vi "Calibration AE.vi"(7 "Command":T1, 8 "error in (no error)":errorcluster, 11 "Inst Details In":string[][](array[string])) -> (0 "error out":errorcluster, 2 "Calibration Due Msg?":string[](array[string]), 3 "Inst Details Out":string[][](array[string]))   [LabVIEW 2016, in "Calibration.lvlib"]
uses:
  Calibration.lvlib
  Calibration Command.ctl
  User Interface/Create Path Command.ctl
  User Interface/User Interface.lvlib
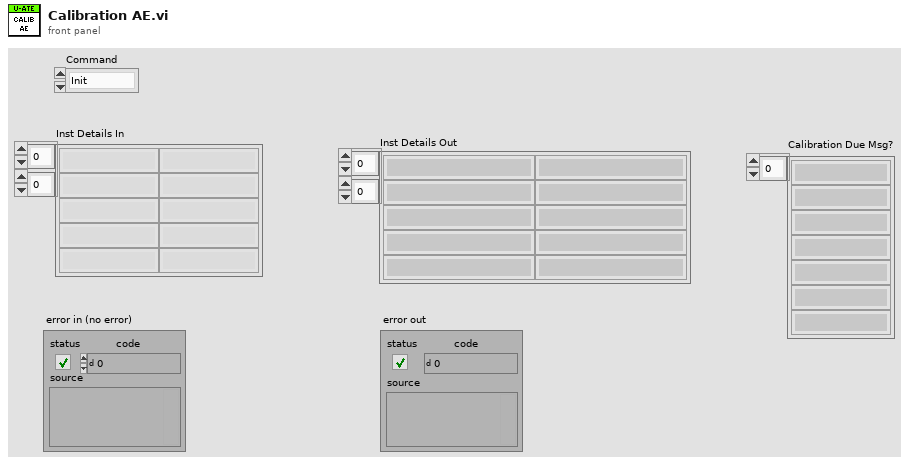
[diagram p1: front panel]
types:
  T1 = typedef "Calibration.lvlib/Calibration Command.ctl" = enum16{"Init", "Read", "Write", "Check Calibration", "Close"}
  T2 = typedef "User Interface.lvlib/Create Path Command.ctl" = enum16{"Authentication", "Hardware", "Configuration", "Calibration", "Instrument", "Test Description", "Data", "Report", "Action log", "Error Log"}
  T3 = enum16{"open", "open or create", "create or replace", "create", "open (read-only)"}
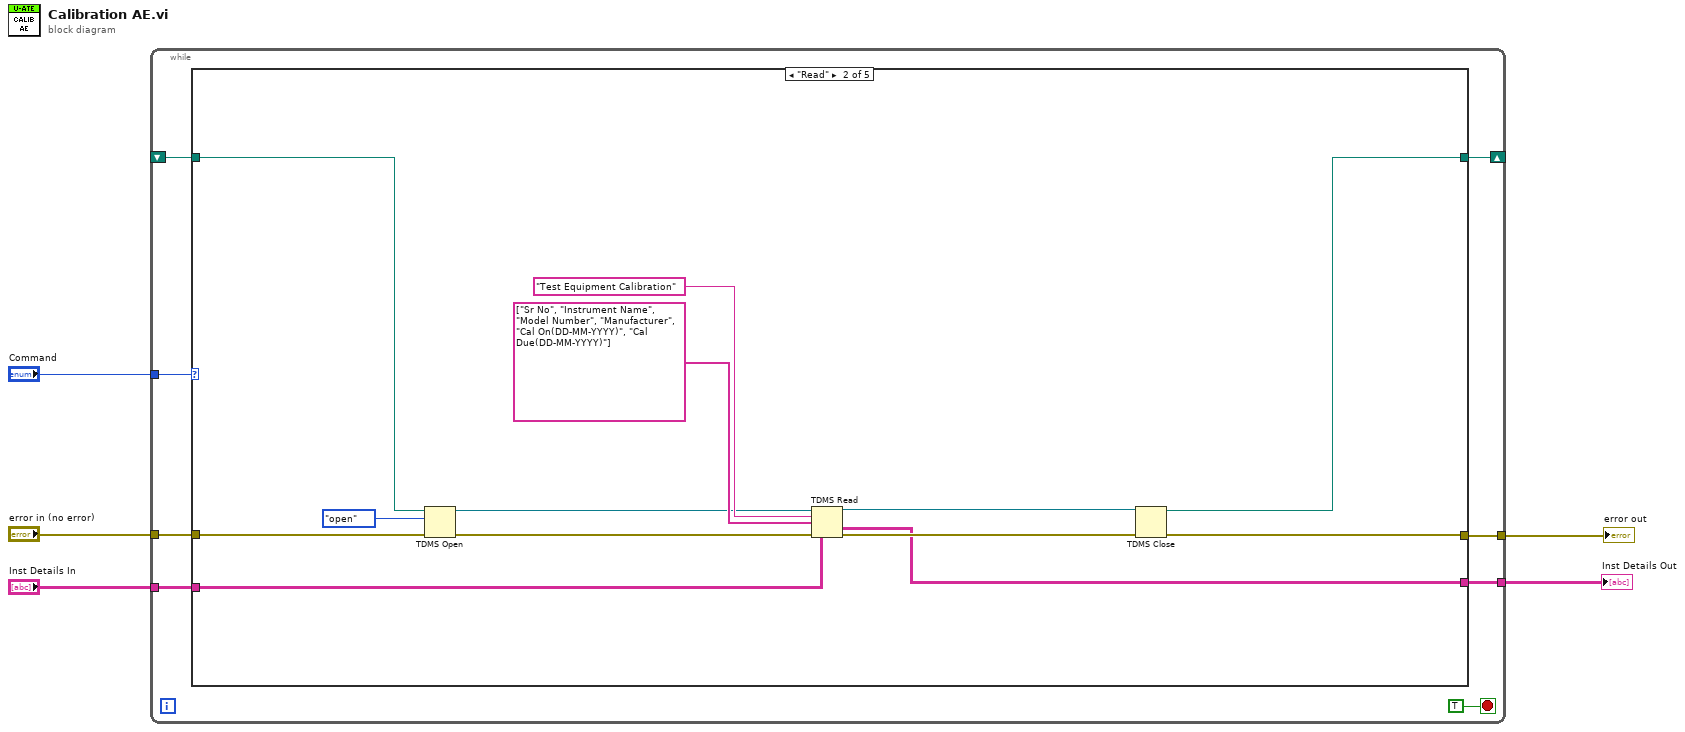
[diagram p0: block diagram]
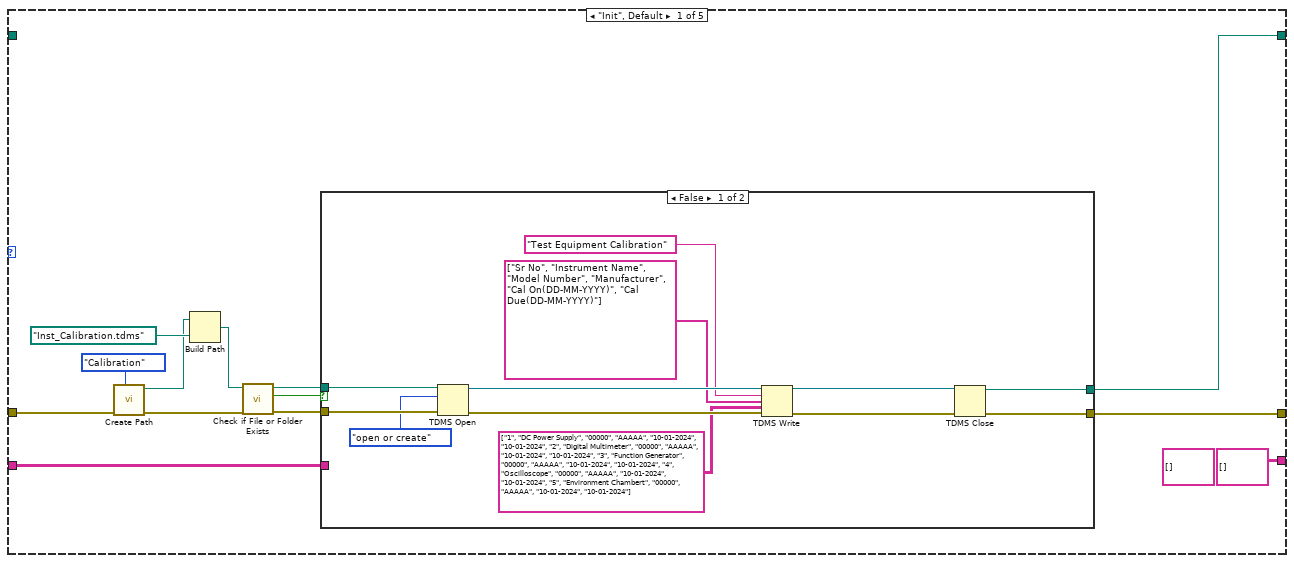
[diagram p2: hidden frame]
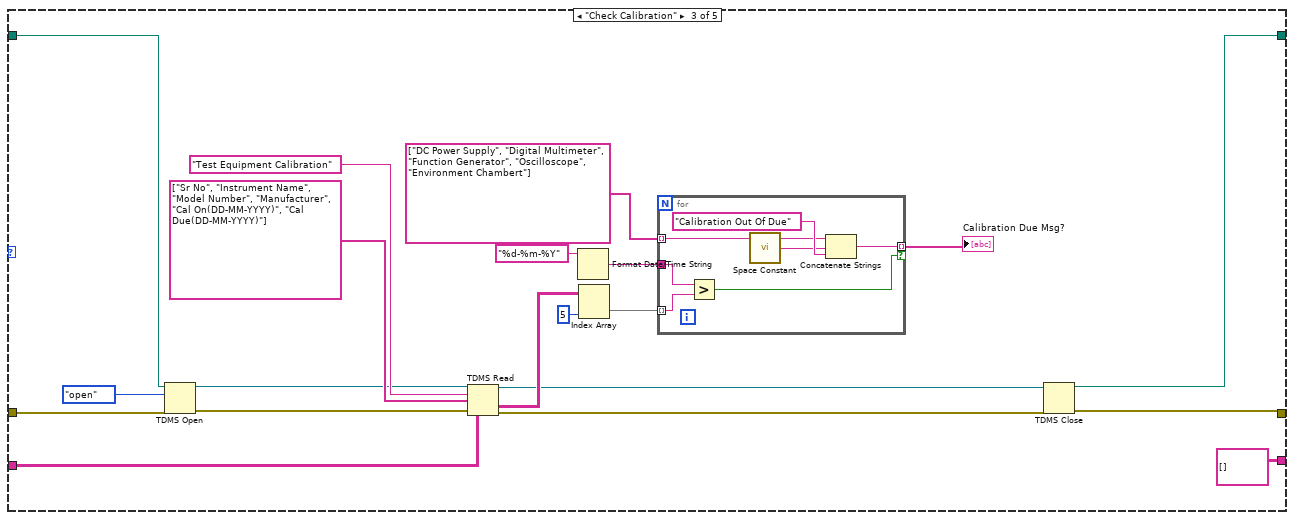
[diagram p4: hidden frame]
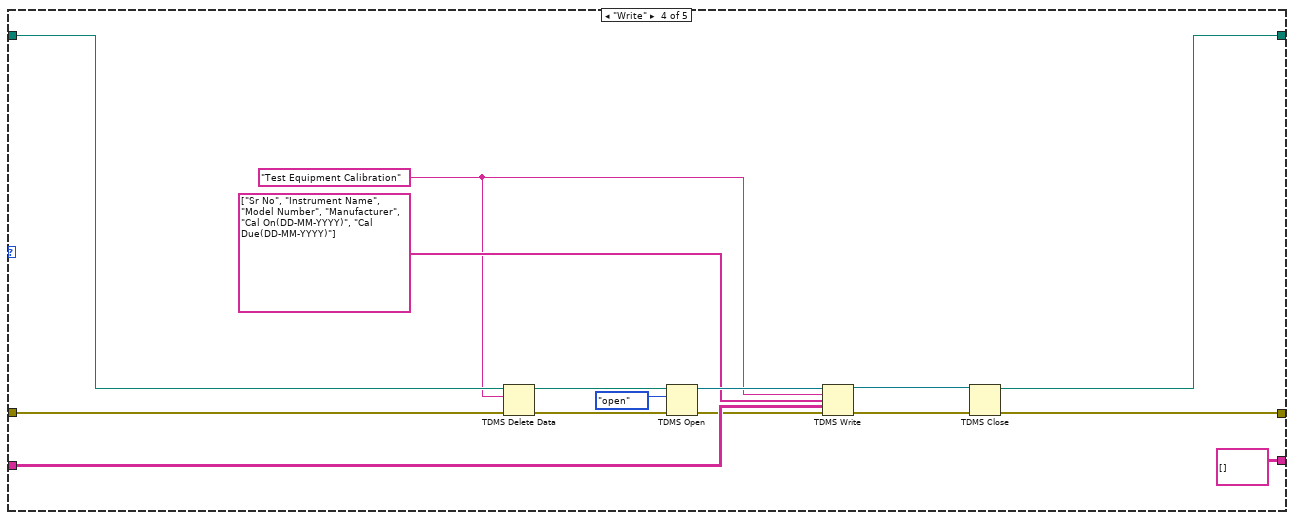
[diagram p5: hidden frame]
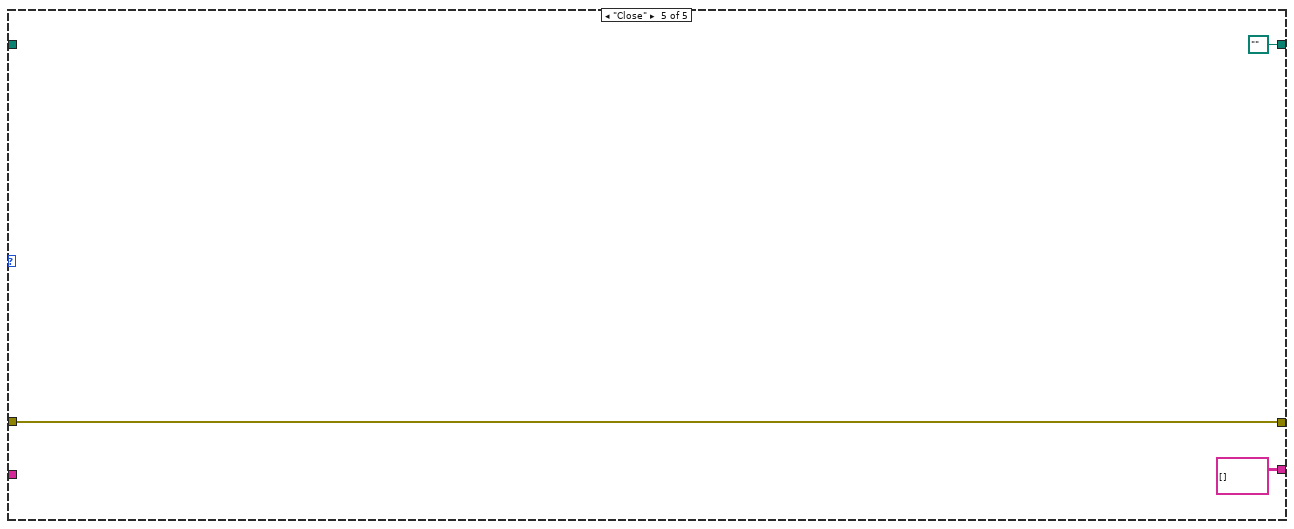
[diagram p6: hidden frame]
diagram:
  n1 = while {
    tunnel: "error in (no error)" -> [w12]
    tunnel: "Inst Details In" -> [w10]
    tunnel: [w9] -> w2
    tunnel: "Command" -> [w11]
    tunnel: [w8] -> w1
    shift-right: [w7] -> _
    shift-left: _ -> [w6]
    stop <- TRUE stop-if-true
    n2 = case shown="\"Read\"" w11 {
      tunnel: w12 -> [w26 w53 w72 w87 w98]
      tunnel: w10 -> [w20 w50 w68 w94 _]
      tunnel: [w19 w43 w56 w90 w98] -> w9
      tunnel: [string[][] [] ("Inst Details In") w48 string[][] [] ("Inst Details In") string[][] [] ("Inst Details In") string[][] [] ("Inst Details In")] -> w8
      tunnel: [w17 w41 w55 w88 path "" ("file path out")] -> w7
      tunnel: w6 -> [_ w46 w71 w86 _]
      frame "Init", Default {
        (unwired) string[][] [] ("Inst Details In")
        n3 = call "Create Path.vi"("Path Command"=Create_Path_Command."Calibration", "error in (no error)"=w26) -> ("error out"=w16:errorcluster, "created path"=w14:path)  [unwired: 8 in]
        n4 = Build Path(base path=w14, name or relative path=path "Inst_Calibration.tdms") -> (appended path=w24:path)
        n5 = call <vilib>:"Check if File or Folder Exists.vi"("error in (no error)"=w16, "path"=w24) -> ("error out"=w23:errorcluster, "file or folder exists?"=w22:bool, "dup path"=w21:path)  [unwired: 7 in]
        n6 = case shown="False" w22 {
          tunnel: w23 -> [w38 w40]
          tunnel: w21 -> [w37 w39]
          tunnel: w20 -> [_ _]
          tunnel: [w28 w40] -> w19
          tunnel: [w29 w39] -> w17
          frame False {
            n7 = TDMS Open(8:w38, 10:T3."open or create" ("operation (0:open)"), 11:w37) -> (0:w34:errorcluster, 3:w35:refnum<k34>)  [unwired: 4 in]
            n8 = TDMS Write(0:w35, 5:"Test Equipment Calibration" ("group name in (Untitled)"), 7:string[] ["Sr No", "Instrument Name", "Model Number", "Manufacturer", "Cal On(DD-MM-YYYY)", "Cal Due(DD-MM-YYYY)"], 9:string[][] [["1", "DC Power Supply", "00000", "AAAAA", "10-01-2024", "10-01-2024"], ["2", "Digital Multimeter", "00000", "AAAAA", "10-01-2024", "10-01-2024"], ["3", "Function Generator", "00000", "AAAAA", "10-01-2024", "10-01-2024"], ["4", "Oscilloscope", "00000", "AAAAA", "10-01-2024", "10-01-2024"], ["5", "Environment Chambert", "00000", "AAAAA", "10-01-2024", "10-01-2024"]], 11:w34) -> (4:w31:refnum<k34>, 15:w30:errorcluster)  [unwired: 1 in, 2 out]
            n9 = TDMS Close(8:w30, 11:w31) -> (0:w28:errorcluster, 3:w29:path)
          }
          frame True {
          }
        }
      }
      frame "Read" {
        n10 = TDMS Open(8:w53, 10:T3."open" ("operation (0:open)"), 11:w46) -> (0:w47:errorcluster, 3:w44:refnum<k34>)  [unwired: 4 in]
        n11 = TDMS Read(0:w44, 5:"Test Equipment Calibration" ("group name in (Untitled)"), 7:string[] ["Sr No", "Instrument Name", "Model Number", "Manufacturer", "Cal On(DD-MM-YYYY)", "Cal Due(DD-MM-YYYY)"], 11:w47, 12:w50) -> (4:w42:refnum<k34>, 10:w48:string[][], 15:w49:errorcluster)  [unwired: 3 in, 3 out]
        n12 = TDMS Close(8:w49, 11:w42) -> (0:w43:errorcluster, 3:w41:path)
      }
      frame "Check Calibration" {
        n13 = TDMS Open(8:w72, 10:T3."open" ("operation (0:open)"), 11:w71) -> (0:w67:errorcluster, 3:w66:refnum<k34>)  [unwired: 4 in]
        n14 = TDMS Read(0:w66, 5:"Test Equipment Calibration" ("group name in (Untitled)"), 7:string[] ["Sr No", "Instrument Name", "Model Number", "Manufacturer", "Cal On(DD-MM-YYYY)", "Cal Due(DD-MM-YYYY)"], 11:w67, 12:w68) -> (4:w58:refnum<k34>, 10:w65:string[][], 15:w57:errorcluster)  [unwired: 3 in, 3 out]
        n15 = Format Date/Time String(time format string (%c)="%d-%m-%Y") -> (date/time string=w61:string)  [unwired: 2 in]
        n16 = Index Array(array=w65, index (col)=5 ("disabled index (col)")) -> (element=w63:string[])  [unwired: 1 in]
        n17 = for {
          tunnel: w63 -> [w79] mode=indexing
          tunnel: w61 -> [w80]
          tunnel: string[] ["DC Power Supply", "Digital Multimeter", "Function Generator", "Oscilloscope", "Environment Chambert"] -> [w76] mode=indexing
          tunnel: [w75] -> w59 mode=indexing if=w74
          n18 = Greater?(x=w80, y=w79) -> (0:w74:bool)
          n19 = call <vilib>:"Space Constant.vi"() -> ("String"=w77:string)
          n20 = Concatenate Strings(w76, w77, "Calibration Out Of Due" ("string")) -> (w75:string)
        }
        "Calibration Due Msg?" <- w59
        n21 = TDMS Close(8:w57, 11:w58) -> (0:w56:errorcluster, 3:w55:path)
      }
      frame "Write" {
        w81 = "Test Equipment Calibration" ("group name in (Untitled)")
        n22 = TDMS Delete Data(8:w87, 10:w81, 11:w86) -> (0:w84:errorcluster, 3:w83:path)  [unwired: 4 in]
        n23 = TDMS Open(8:w84, 10:T3."open" ("operation (0:open)"), 11:w83) -> (0:w82:errorcluster, 3:w91:refnum<k34>)  [unwired: 4 in]
        n24 = TDMS Write(0:w91, 5:w81, 7:string[] ["Sr No", "Instrument Name", "Model Number", "Manufacturer", "Cal On(DD-MM-YYYY)", "Cal Due(DD-MM-YYYY)"], 9:w94, 11:w82) -> (4:w89:refnum<k34>, 15:w95:errorcluster)  [unwired: 1 in, 2 out]
        n25 = TDMS Close(8:w95, 11:w89) -> (0:w90:errorcluster, 3:w88:path)
      }
      frame "Close" {
      }
    }
  }
  "error out" <- w2
  "Inst Details Out" <- w1
